vi "Stop.vi"(8 "error in":errorcluster, 11 "PCAN-USB Read-Write Raw CAN Frame Strategy in":refnum<class "PCAN-USB Base Strategy.lvclass">) -> (0 "error out":errorcluster, 3 "PCAN-USB Read-Write Raw CAN Frame Strategy out":refnum<class "PCAN-USB Base Strategy.lvclass">)   [LabVIEW 2024, in "PCAN-USB Base Strategy.lvclass"]
uses:
  PCAN-USB Base Strategy.lvclass
  PCAN-USB Base Strategy.lvclass/PCAN-USB Base Strategy.ctl
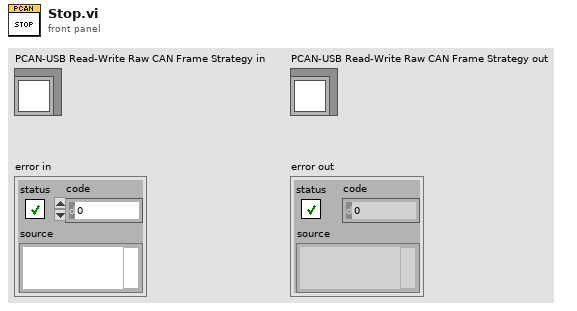
[diagram p1: front panel]
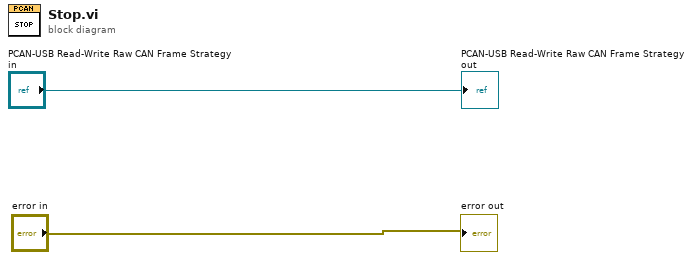
[diagram p0: block diagram]
diagram:
  "error out" <- "error in"
  "PCAN-USB Read-Write Raw CAN Frame Strategy out" <- "PCAN-USB Read-Write Raw CAN Frame Strategy in"
